vi "Configure Module.vi"(8 "error in (no error)":errorcluster, 10 "IOV ref in":refnum<k21>, 11 "9237 in":refnum<class "9237.lvclass">) -> (0 "error out":errorcluster, 2 "IOV ref out":refnum<k21>, 3 "9237 out":refnum<class "9237.lvclass">)   [LabVIEW 2017, in "Modules.lvlib" / "9237.lvclass"]
uses:
  9237.lvclass
  9237.lvclass/9237.ctl
  <resource>/objmgr/cRIO.rc
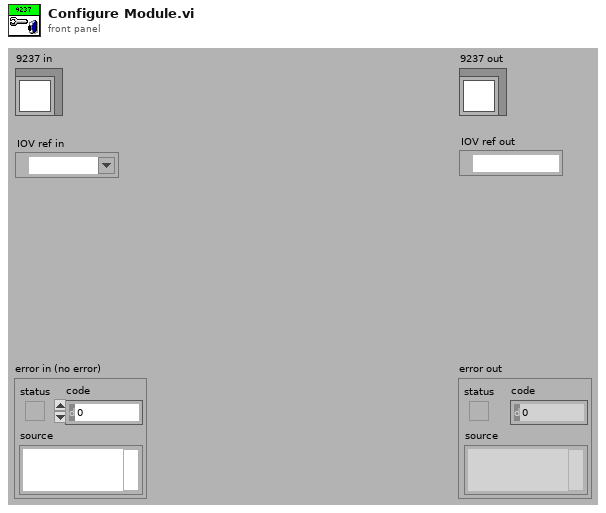
[diagram p1: front panel]
types:
  T1 = typedef "Modules.lvlib/9237.lvclass/_nicrio_cRIO-923x_ExcitationVoltageRing.ctl" = u8
  T2 = typedef "Modules.lvlib/9237.lvclass/Data rate.ctl" = u32
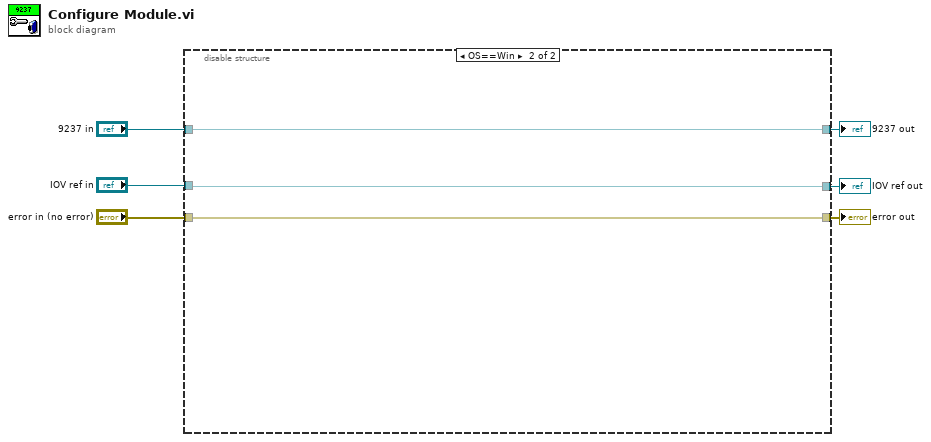
[diagram p0: block diagram]
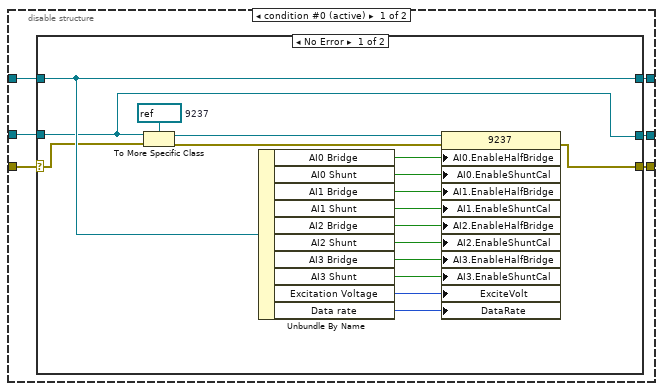
[diagram p2: hidden frame]
diagram:
  n1 = disable-structure shown="OS==Win" {
    disable-tunnel: "error in (no error)" -> [w12 w35]
    disable-tunnel: [w11 w35] -> w5
    disable-tunnel: "9237 in" -> [w10 w33]
    disable-tunnel: [w9 w33] -> w3
    disable-tunnel: "IOV ref in" -> [w8 w34]
    disable-tunnel: [w7 w34] -> w1
    frame condition #0 (active) {
      n2 = case shown="No Error" w12 {
        selector: w12 -> [w19 w32]
        tunnel: [w17 w32] -> w11
        tunnel: [w29 w31] -> w9
        tunnel: w10 -> [w29 w31]
        tunnel: w8 -> [w15 w30]
        tunnel: [w15 w30] -> w7
        frame No Error {
          w20 = refnum<k21> refnum  # 9237
          n3 = To More Specific Class(target class=w20, reference=w15, error in=w19) -> (specific class reference=w14:refnum<k21>, error out=w18:errorcluster)
          n4 = Unbundle By Name(w29) -> ("AI0 Bridge"=w28:bool, "AI0 Shunt"=w27:bool, "AI1 Bridge"=w26:bool, "AI1 Shunt"=w25:bool, "AI2 Bridge"=w24:bool, "AI2 Shunt"=w23:bool, "AI3 Bridge"=w22:bool, "AI3 Shunt"=w21:bool, "Excitation Voltage"=w16:T1, "Data rate"=w13:T2)
          n5 = property class="9237"(reference=w14, error in=w18, "AI0.EnableHalfBridge"=w28, "AI0.EnableShuntCal"=w27, "AI1.EnableHalfBridge"=w26, "AI1.EnableShuntCal"=w25, "AI2.EnableHalfBridge"=w24, "AI2.EnableShuntCal"=w23, "AI3.EnableHalfBridge"=w22, "AI3.EnableShuntCal"=w21, "ExciteVolt"=w16, "DataRate"=w13) -> (error out=w17:errorcluster)  [unwired: 1 out]
        }
        frame Error {
        }
      }
    }
    frame condition #1 {
    }
  }
  "error out" <- w5
  "9237 out" <- w3
  "IOV ref out" <- w1
